vi "Get ROIAndBin.vi"(8 "error in (no error)":errorcluster, 11 "TLCamera reference in":refnum<k24>) -> (0 "error out":errorcluster, 1 "Region of Interest":T1={"Origin - X"=0, "Origin - Y"=0, "Width"=1392, "Height"=1040}, 2 "Binning":T2, 3 "TLCamera reference out":refnum<k24>)   [LabVIEW 2019]
uses:
  C:/Users/jleeman/git_repos/CAxis_Machine/C-Axis LabView Controller/Library_X64/Thorlabs.TSI.TLCameraInterfaces.dll
  Library_X64/Thorlabs.TSI.TLCameraInterfaces.dll
  Thor_Controls/Binning.ctl
  Thor_Controls/Region of Interest.ctl
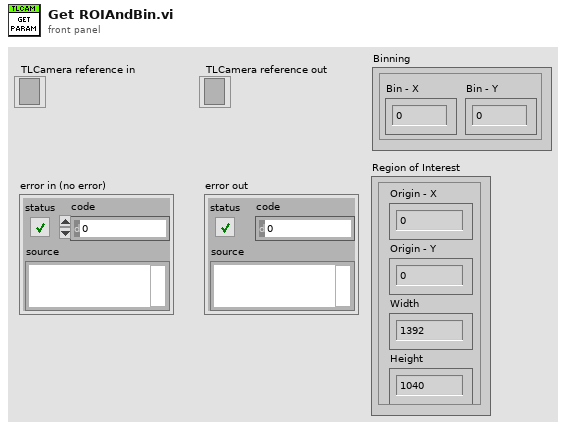
[diagram p1: front panel]
types:
  T1 = typedef "Region of Interest.ctl" = cluster{"Origin - X":u32, "Origin - Y":u32, "Width":u32, "Height":u32}
  T2 = typedef "Binning.ctl" = cluster{"Bin - X":u32, "Bin - Y":u32}
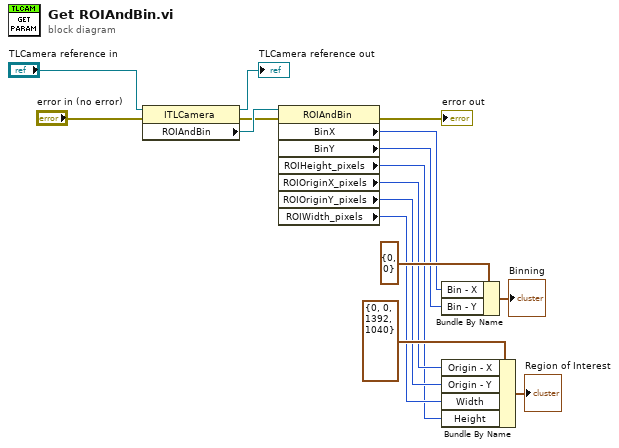
[diagram p0: block diagram]
diagram:
  n1 = property class="ITLCamera"(reference="TLCamera reference in", error in="error in (no error)") -> (reference out=→"TLCamera reference out":refnum<k24>, error out=w12:errorcluster, "ROIAndBin"=w13:refnum<k24>)
  n2 = property class="ROIAndBin"(reference=w13, error in=w12) -> (error out=→"error out":errorcluster, "BinX"=w10:u32, "BinY"=w9:u32, "ROIHeight_pixels"=w4:u32, "ROIOriginX_pixels"=w7:u32, "ROIOriginY_pixels"=w6:u32, "ROIWidth_pixels"=w5:u32)  [unwired: 1 out]
  n3 = Bundle By Name(cluster=T2 {"Bin - X"=0, "Bin - Y"=0} ("Binning"), "Bin - X"=w10, "Bin - Y"=w9) -> (→"Binning":T2)
  n4 = Bundle By Name(cluster=T1 {"Origin - X"=0, "Origin - Y"=0, "Width"=1392, "Height"=1040} ("Region of Interest"), "Origin - X"=w7, "Origin - Y"=w6, "Width"=w5, "Height"=w4) -> (→"Region of Interest":T1)
